vi "fftfreq.vi"() -> ()   [LabVIEW 2020]
panel:
  out "val":fxp<+,64,48>
  out "n*d":fxp<+,32,16>
  out "f":fxp<+/-,32,16>[](array[numeric])
  out "size(s)":i32
  out "output array":fxp<+/-,32,32>[](array[numeric])
  out "p 2":fxp<+/-,32,32>[](array[numeric])
  out "p1":fxp<+/-,32,32>[](array[numeric])
  out "N":fxp<+/-,18,17>
  in  "n":fxp<+,32,16>
  in  "s (sample rate)":fxp<+,32,16>
  # "n=512"
  # "s=51200"
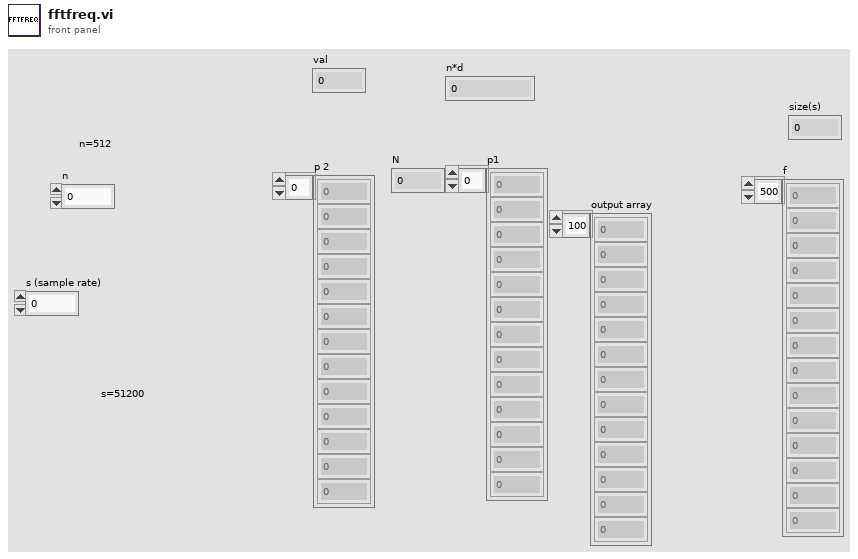
[diagram p1: front panel]
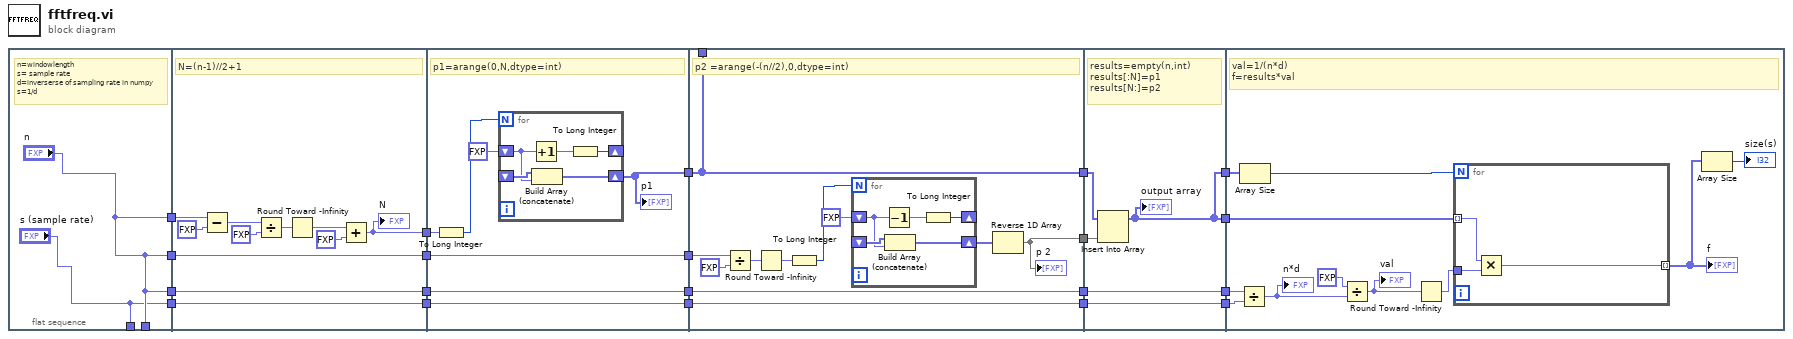
[diagram p0: block diagram]
diagram:
  n1 = flat-sequence {
    tunnel: ["n"] -> w20
    tunnel: ["s (sample rate)"] -> _
    tunnel: ["n"] -> _
    tunnel: ["s (sample rate)"] -> w19
    tunnel: ["n"] -> w18
    tunnel: ["n"] -> w17
    tunnel: [w27] -> w16
    tunnel: w20 -> [w26]
    tunnel: w19 -> [w25]
    tunnel: [w25] -> w15
    tunnel: w18 -> [w24]
    tunnel: [w24] -> w14
    tunnel: w17 -> [w23]
    tunnel: [w23] -> w13
    tunnel: w16 -> [w39]
    tunnel: [w37] -> w12
    tunnel: w15 -> [w36]
    tunnel: [w36] -> w11
    tunnel: w14 -> [w35]
    tunnel: [w35] -> w10
    tunnel: w13 -> [w34]
    tunnel: [w34] -> w9
    tunnel: [w50] -> w8
    tunnel: [w46] -> _
    tunnel: w12 -> [w46]
    tunnel: w11 -> [w49]
    tunnel: [w49] -> w7
    tunnel: w10 -> [w48]
    tunnel: w9 -> [w47]
    tunnel: [w47] -> w6
    tunnel: [w46] -> w5
    tunnel: w8 -> [w66]
    tunnel: w7 -> [w65]
    tunnel: [w65] -> w4
    tunnel: [w64] -> w3
    tunnel: [w64] -> w2
    tunnel: w6 -> [w63]
    tunnel: [w63] -> w1
    tunnel: w5 -> [w62]
    tunnel: w4 -> [w72]
    tunnel: w3 -> [w71]
    tunnel: w2 -> [w70]
    tunnel: w1 -> [w69]
    frame #0 {
      # "n=windowlength\ns= sample rate\nd=inverserse of sampling rate in numpy\ns=1/d"
    }
    frame #1 {
      # "N=(n-1)//2+1"
      n2 = Subtract(x=w26, y=fxp<+,1,1> 1.0) -> (x-y=w31:fxp<+/-,33,17>)
      n3 = Divide(x=w31, y=fxp<+,1,2> 2.0) -> (x/y=w32:fxp<+/-,34,16>)
      n4 = Round Toward -Infinity(1:w32) -> (0:w33:fxp<+/-,16,16>)
      n5 = Add(x=w33, y=fxp<+,1,1> 1.0) -> (x+y=w27:fxp<+/-,18,17>)
      "N" <- w27
    }
    frame #2 {
      # "p1=arange(0,N,dtype=int)"
      n6 = To Long Integer(number=w39) -> (32bit integer=w40:i32)
      n7 = for {
        N: w40 -> [_]
        shift-right: [w41] -> _
        shift-left: fxp<+,1,1> 0.0 -> [w43]
        shift-right: [w44] -> w37
        shift-left: _ -> [w45]
        n8 = Increment(x=w43) -> (x+1=w42:fxp<+/-,33,33>)
        n9 = Build Array (concatenate)(w45, w43) -> (w44:fxp<+/-,32,32>[])
        n10 = To Long Integer(number=w42) -> (32bit integer=w41:i32)
      }
      "p1" <- w37
    }
    frame #3 {
      # "p2 =arange(-(n//2),0,dtype=int)"
      n11 = Divide(x=w48, y=fxp<+,1,2> 2.0) -> (x/y=w53:fxp<+,33,15>)
      n12 = Round Toward -Infinity(1:w53) -> (0:w55:fxp<+,15,15>)
      n13 = To Long Integer(number=w55) -> (32bit integer=w54:i32)
      n14 = for {
        N: w54 -> [_]
        shift-right: [w57] -> _
        shift-left: fxp<+,1,1> 0.0 -> [w59]
        shift-right: [w60] -> w56
        shift-left: _ -> [w61]
        n15 = Decrement(x=w59) -> (x-1=w58:fxp<+/-,33,33>)
        n16 = Build Array (concatenate)(w61, w59) -> (w60:fxp<+/-,32,32>[])
        n17 = To Long Integer(number=w58) -> (32bit integer=w57:i32)
      }
      n18 = Reverse 1D Array(array=w56) -> (reversed array=w50:fxp<+/-,32,32>[])
      "p 2" <- w50
    }
    frame #4 {
      # "results=empty(n,int)\nresults[:N]=p1\nresults[N:]=p2"
      n19 = Insert Into Array(array=w62, new element=w66) -> (w64:fxp<+/-,32,32>[])  [unwired: 1 in]
      "output array" <- w64
    }
    frame #5 {
      # "val=1/(n*d)\nf=results*val"
      n20 = Divide(x=w69, y=w72) -> (x/y=w75:fxp<+,64,32>)
      "n*d" <- w75
      n21 = Array Size(array=w71) -> (size(s)=w74:i32)
      n22 = Divide(x=fxp<+,32,32> 1.0, y=w75) -> (x/y=w76:fxp<+,32,16>)
      "val" <- w76
      n23 = Round Toward -Infinity(1:w76) -> (0:w77:fxp<+,16,16>)
      n24 = for {
        N: w74 -> [_]
        tunnel: w77 -> [w80]
        tunnel: [w78] -> w68 mode=indexing
        tunnel: w70 -> [w79] mode=indexing
        n25 = Multiply(x=w79, y=w80) -> (x*y=w78:fxp<+/-,32,16>)
      }
      "f" <- w68
      n26 = Array Size(array=w68) -> (size(s)=→"size(s)":i32)
    }
  }
